vi "Open.vi"(7 "IPstr":string, 8 "error in (no error)":errorcluster, 9 "timeout ms (60000)":i32=60000, 10 "port":u16) -> (0 "error out":errorcluster, 3 "connection ID":refnum<k16>)   [LabVIEW 2018, in "Simple UDP Message.lvlib"]
uses:
  Simple UDP Message.lvlib
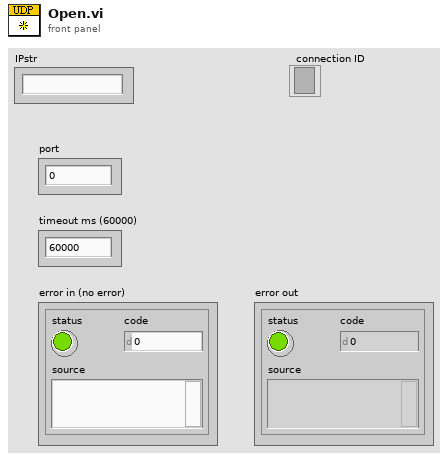
[diagram p1: front panel]
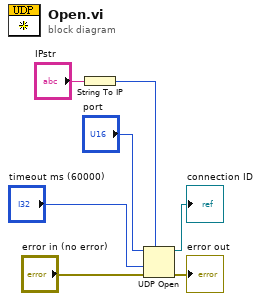
[diagram p0: block diagram]
diagram:
  n1 = String To IP(1:"IPstr") -> (0:w1:u32)
  n2 = UDP Open(7:w1, 8:"error in (no error)", 9:"timeout ms (60000)", 11:"port") -> (port=→"connection ID":refnum<k16>, 0:→"error out":errorcluster)  [unwired: 1 in, 1 out]
